vi "S2C_Exit.vi"(8 "Error In":errorcluster, 11 "S2C-Q":refnum<queue>) -> (0 "Error Out":errorcluster, 3 "Exit?":bool)   [LabVIEW 2015]
doc: "Detects an error and calls the error case to process the error."
uses:
  Globals/S2C_Globals.vi
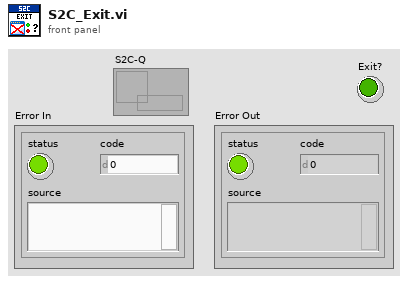
[diagram p1: front panel]
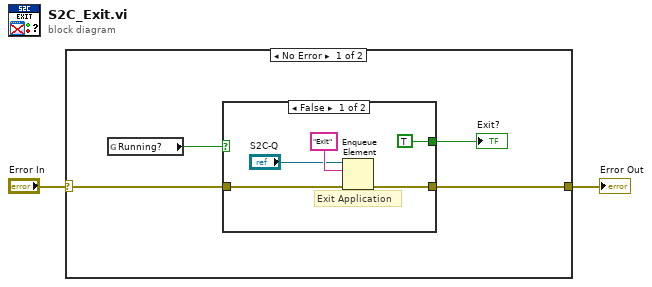
[diagram p0: block diagram]
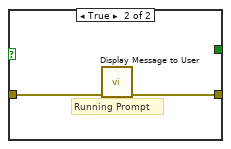
[diagram p2: hidden frame]
diagram:
  n1 = case shown="No Error" "Error In" {
    selector: "Error In" -> [w5 w14]
    tunnel: [w6 w14] -> w1
    frame No Error {
      n2 = global read "S2C_Globals.vi" "Running?"() -> (w4:bool)
      n3 = case shown="False" w4 {
        tunnel: [w10 w12] -> w6
        tunnel: w5 -> [w8 w13]
        tunnel: [TRUE _] -> w3
        frame False {
          # "Exit Application"
          n4 = Enqueue Element(queue="S2C-Q", element="Exit", error in (no error)=w8) -> (error out=w10:errorcluster)  [unwired: 1 in, 2 out]
        }
        frame True {
          # "Running Prompt"
          n5 = call "Display Message to User"("error in (no error)"=w13) -> ("error out"=w12:errorcluster)  [unwired: 9 in, 1 out]
        }
      }
      "Exit?" <- w3
    }
    frame Error {
    }
  }
  "Error Out" <- w1
